vi "Write StreamInfo.vi"(8 "error in (no error)":errorcluster, 10 "StreamInfo":T1, 11 "AODAcq in":refnum<class "AODAcq.lvclass">) -> (0 "error out":errorcluster, 3 "AODAcq out":refnum<class "AODAcq.lvclass">)   [LabVIEW 2014, in "AODAcq.lvclass"]
uses:
  AODAcq.lvclass
  AODAcq.lvclass/AODAcq.ctl
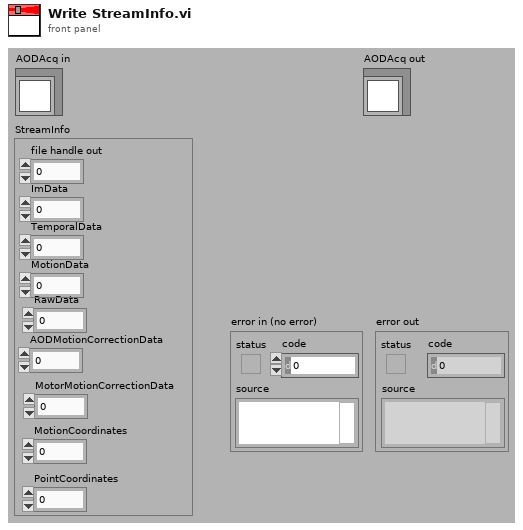
[diagram p1: front panel]
types:
  T1 = cluster{"file handle out":i32, "ImData":i32, "TemporalData":i32, "MotionData":i32, "RawData":i32, "AODMotionCorrectionData":i32, "MotorMotionCorrectionData":i32, "MotionCoordinates":i32, "PointCoordinates":i32}
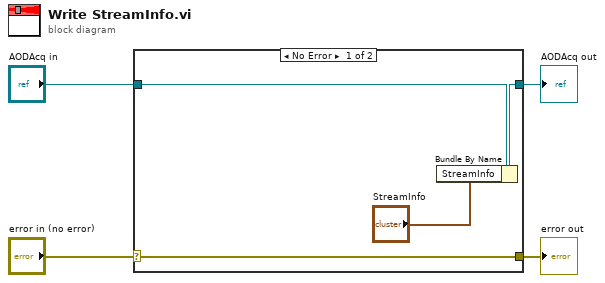
[diagram p0: block diagram]
diagram:
  n1 = case shown="No Error" "error in (no error)" {
    selector: "error in (no error)" -> [w8 w9]
    tunnel: [w8 w9] -> w3
    tunnel: [w6 w10] -> w1
    tunnel: "AODAcq in" -> [w7 w10]
    frame No Error {
      n2 = Bundle By Name(cluster=w7, "StreamInfo"="StreamInfo") -> (w6:refnum<class "AODAcq.lvclass">)
    }
    frame Error {
    }
  }
  "error out" <- w3
  "AODAcq out" <- w1
